vi "Type Conversion.To Double (Boolean).vi"(3 "value in":bool) -> (1 "value out":dbl)   [LabVIEW 2016, in "VeriStand Data.lvlib"]
doc: "Converts the provided values to double floats, preserving the numerical value of the data."
uses:
  VeriStand Data.lvlib
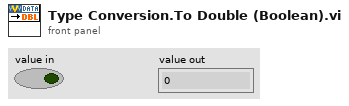
[diagram p1: front panel]
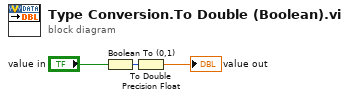
[diagram p0: block diagram]
diagram:
  n1 = Boolean To (0,1)(Boolean="value in") -> (0, 1=w2:i16)
  n2 = To Double Precision Float(number=w2) -> (double precision float=→"value out":dbl)
